vi "TrigNSave.vi"() -> ()   [LabVIEW 2013]
panel:
  in  "Trig Pulse Delay (s)":dbl[](array[numeric])
  in  "Trig Pulse Duration (s)":dbl[](array[numeric])
  in  "Delay between iterations (max exposure, in milliseconds)":i32=2000
  in  "Overwrite":bool
  in  "Save Data":bool
  out "Message":string
  in  "Pulse Energy mJ":dbl=5.0
  in  "File Name":string="log.dat"
  in  "Shot Num":i32
  in  "Shoot Once":bool
  in  "Abort Loop":bool
  out "Looping":bool
  out "Current Shot Number":i32
  in  "Number of shots":i32
  in  "START":bool
  in  "Command":string=":PULSe0:STATe ON"
  in  "Pressure reading mA":dbl=5.0
  in  "Pressure reading bar-a":dbl=1.0
  in  "Pulse Duration fs":dbl=5.0
  in  "Path to Folder":path=path "G:/Développement de Programmes/Programmes/octo-labview/Automatisation Manip Gaz"
  in  "Comments":string
  in  "FLSH":bool
  in  "SEND":bool
  out "error out":errorcluster
  in  "stop":bool
  out "read buffer":string
  in  "error in (no error)":errorcluster
  in  "VISA resource name":refnum<visa-resource-name>="COM1"
  # "Log File"
  # "Loop Control"
  # "BNC 505 Manual Control"
  # "Channel 0"
  # "Channel 1"
  # "Channel 2"
  # "Channel 3"
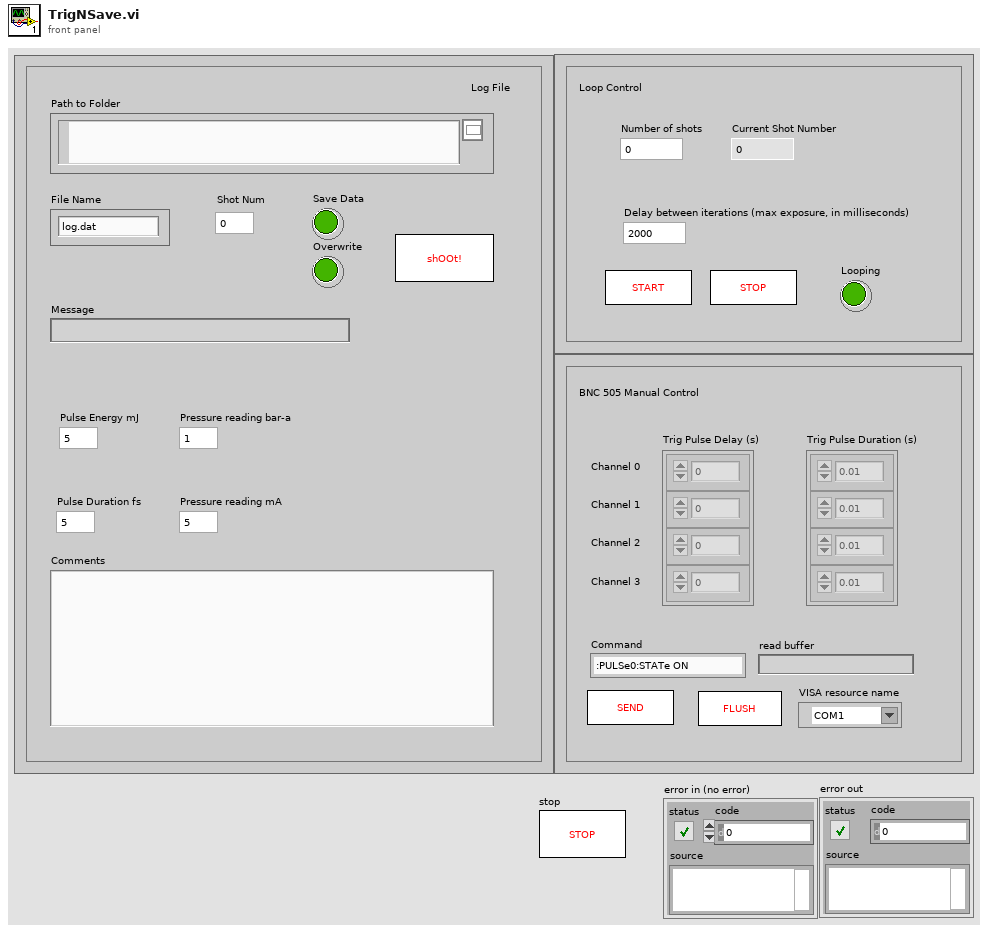
[diagram p1: front panel]
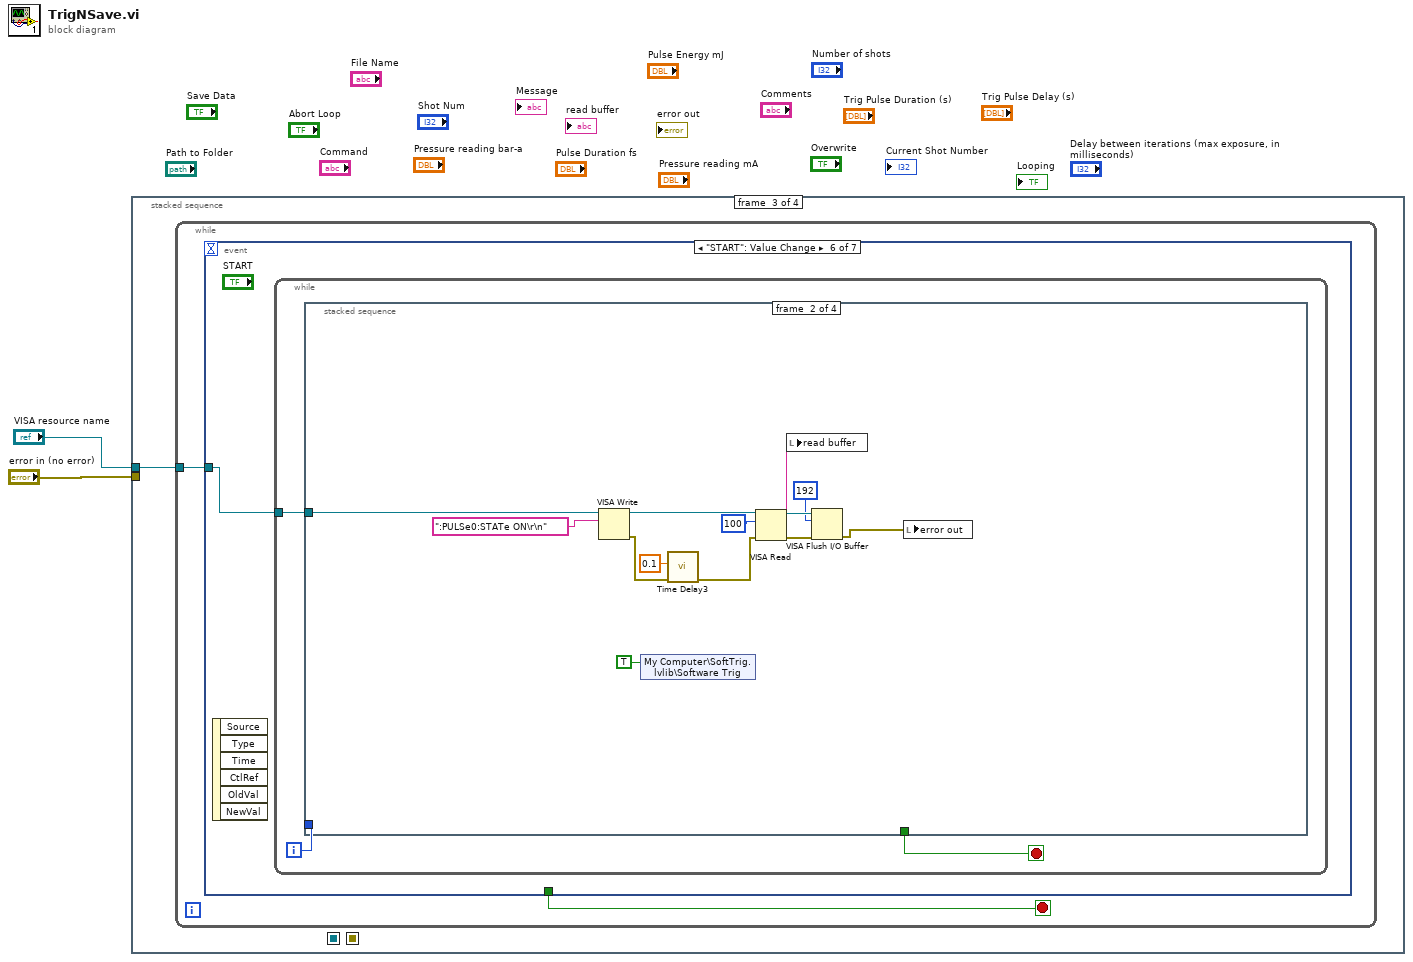
[diagram p0: block diagram]
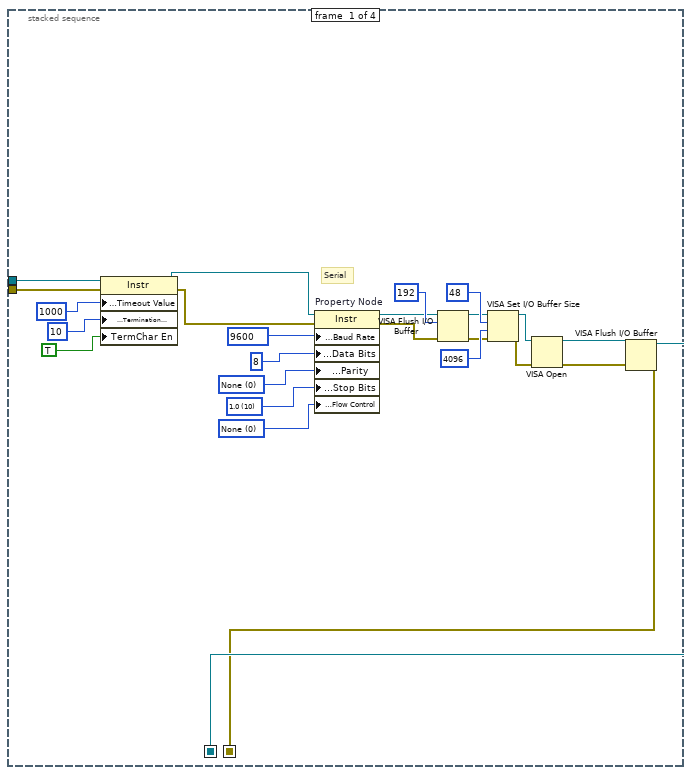
[diagram p2: hidden frame]
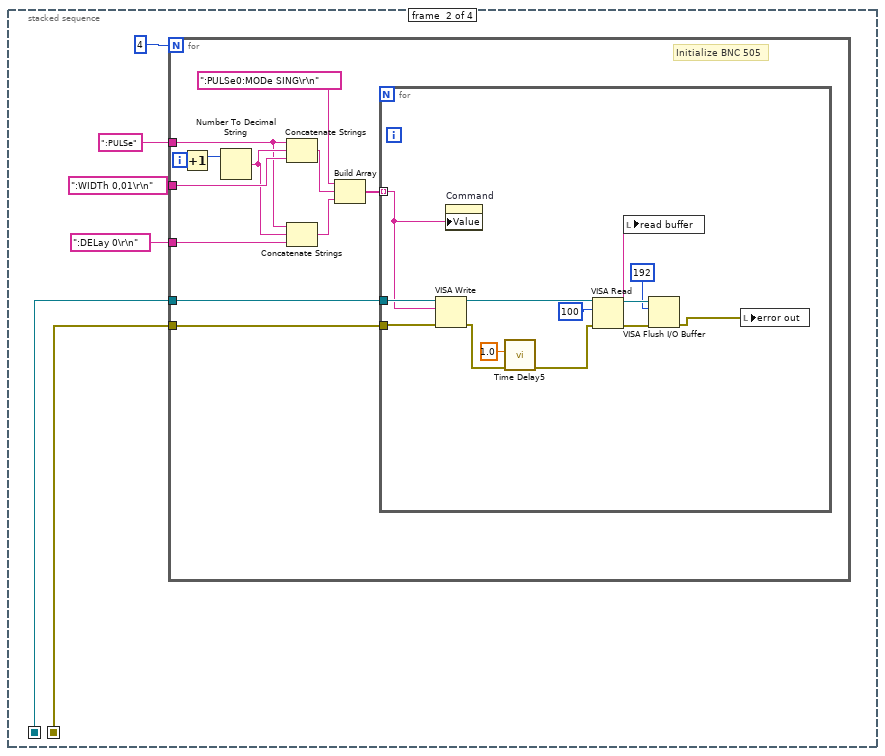
[diagram p3: hidden frame]
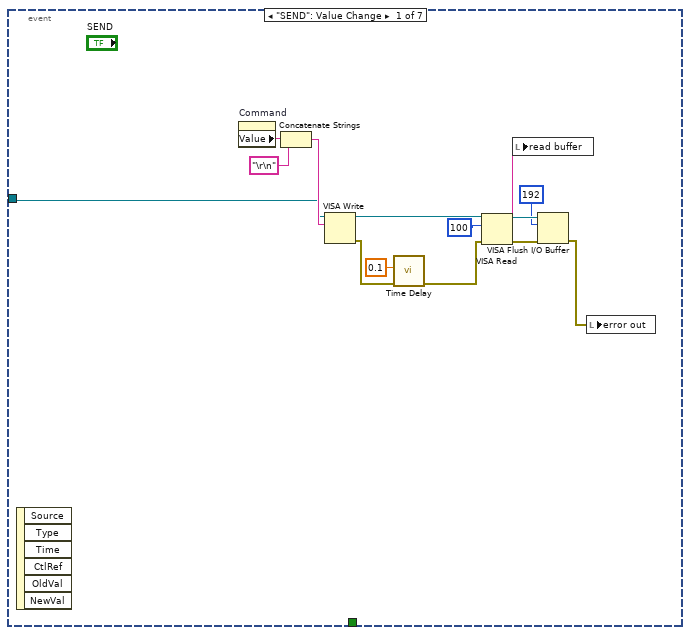
[diagram p4: hidden frame]
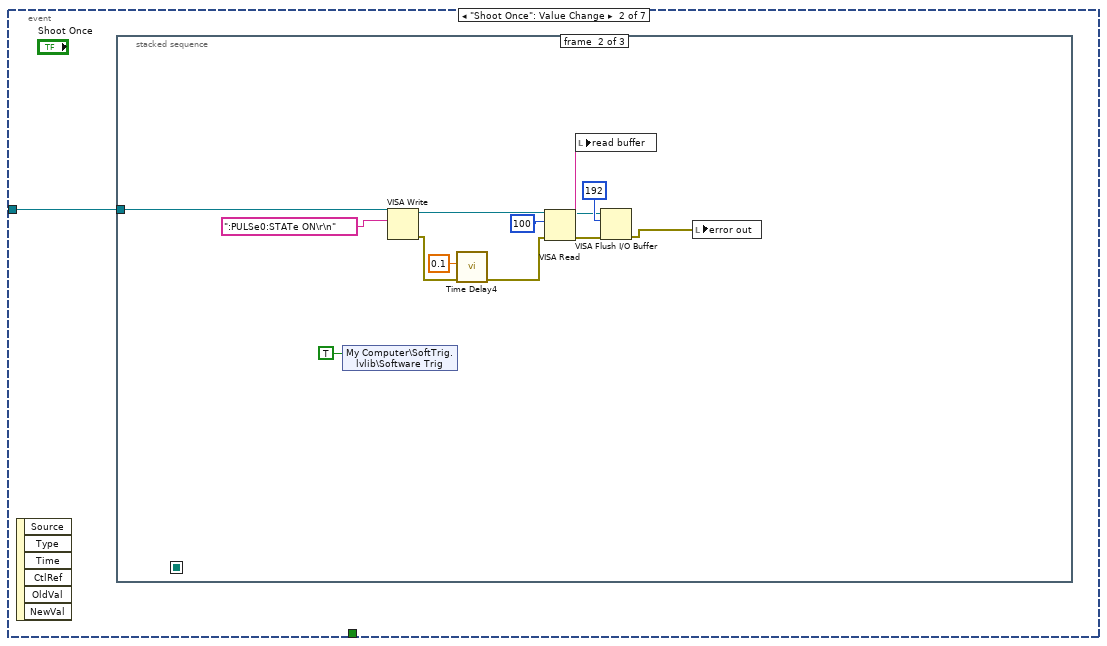
[diagram p5: hidden frame]
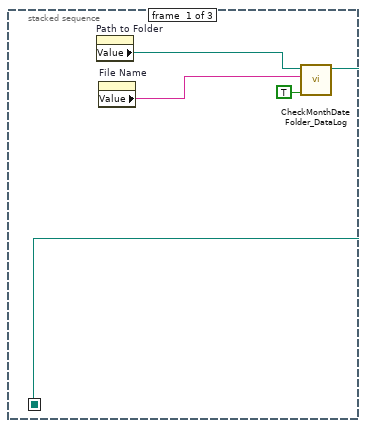
[diagram p6: hidden frame]
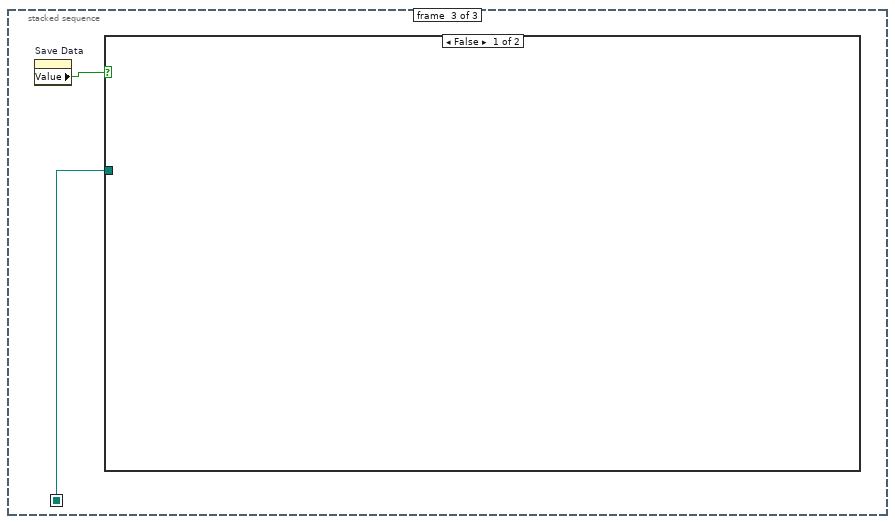
[diagram p7: hidden frame]
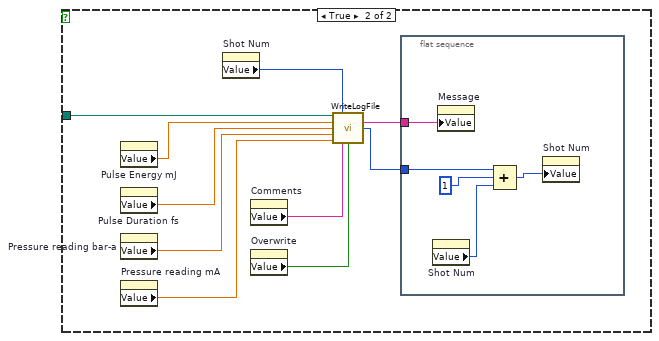
[diagram p8: hidden frame]
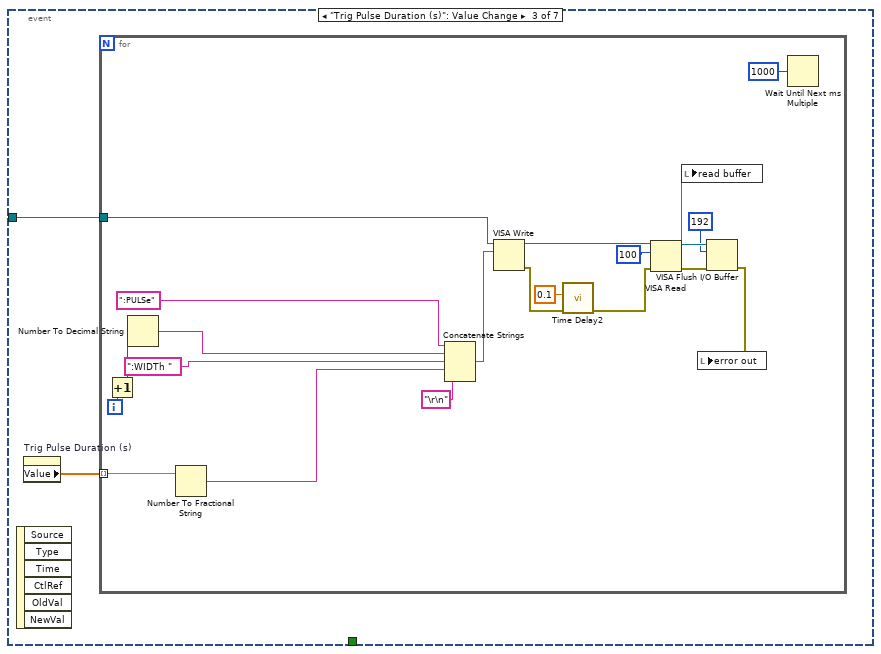
[diagram p9: hidden frame]
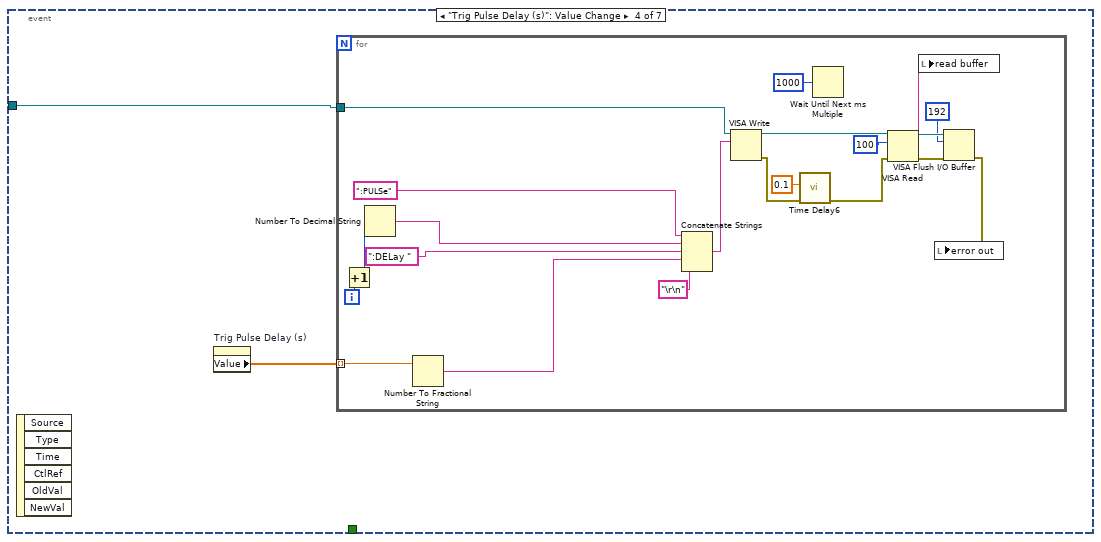
[diagram p10: hidden frame]
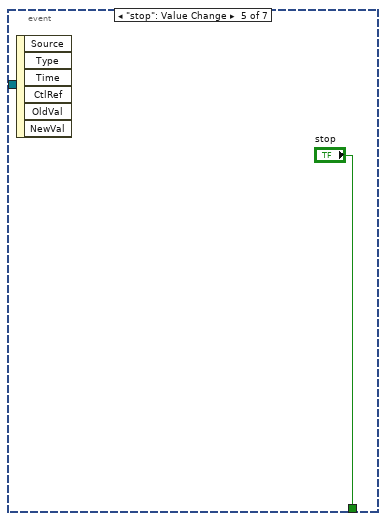
[diagram p11: hidden frame]
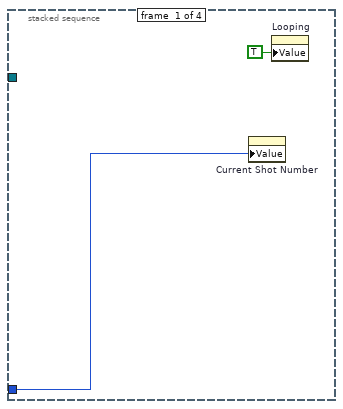
[diagram p12: hidden frame]
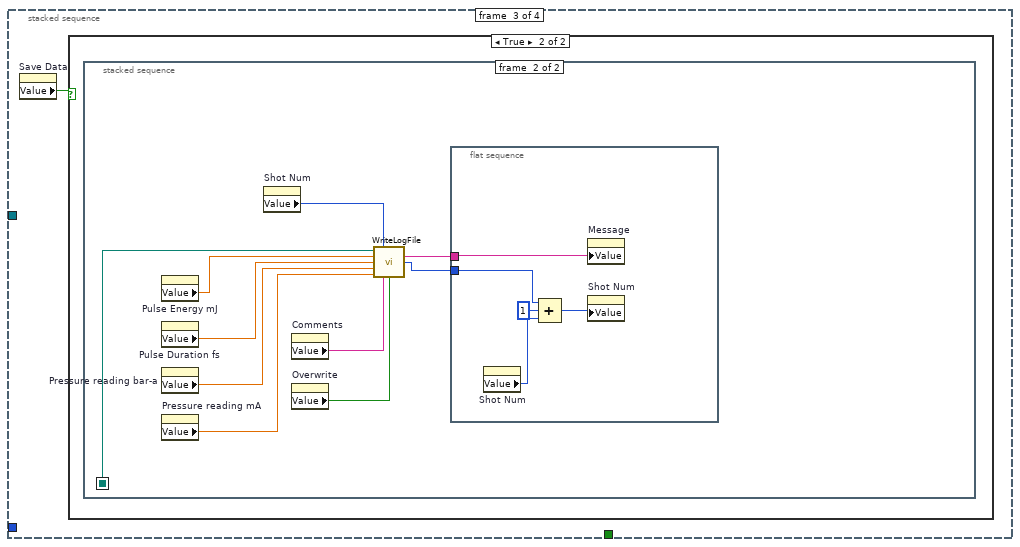
[diagram p13: hidden frame]
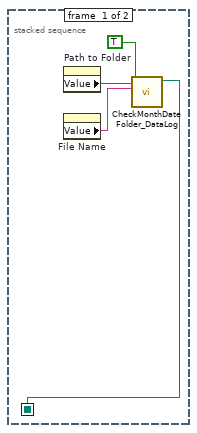
[diagram p15: hidden frame]
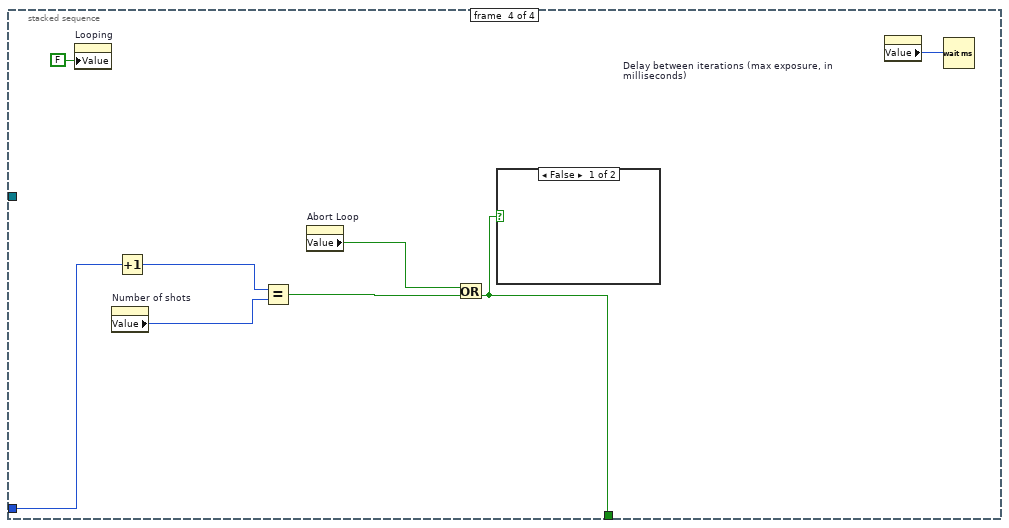
[diagram p16: hidden frame]
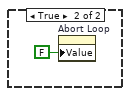
[diagram p17: hidden frame]
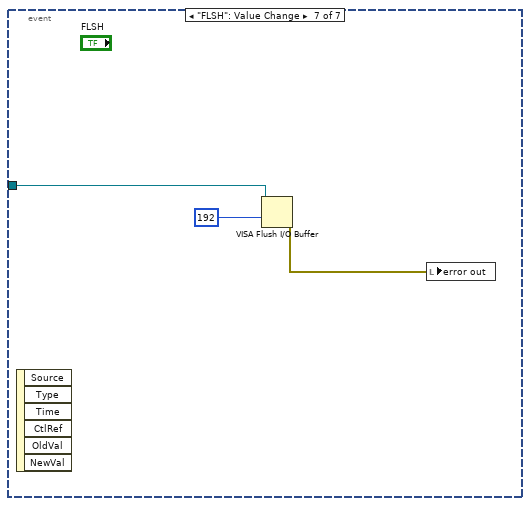
[diagram p18: hidden frame]
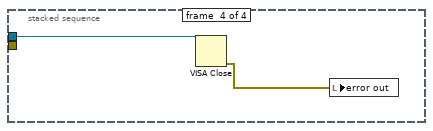
[diagram p19: hidden frame]
diagram:
  n1 = stacked-sequence {
    seq-local: [w4 _ _ _] -> [_ w33 _ _]
    seq-local: [w3 _ _ _] -> [_ w32 _ _]
    tunnel: "error in (no error)" -> [w22 _ _ _]
    tunnel: "VISA resource name" -> [w5 _ w59 w210]
    frame #0 {
      w11 = u32 9600 items=["4800"=4600, "9600"=9600, "19200"=19200, "38400"=38400, "57600"=57600, "115200"=115200] ("Baud Rate (make sure matches instrument)")
      w8 = u16 0 items=["None"=0, "XON/XOFF"=1, "RTS/CTS"=2, "DTR/DSR"=4] ("Serial Settings:Serial Flow Control")
      w19 = u16 10 items=["1.0"=10, "1.5"=15, "2.0"=20] ("Serial Settings:Serial Stop Bits")
      w20 = u16 0 items=["None", "Odd", "Even", "Mark", "Space"] ("Serial Settings:Serial Parity")
      # "Serial"
      n2 = property class="Instr"(reference=w5, error in=w22, "General Settings:Timeout Value"=u32 1000, "Message Based Settings:Termination Character"=u8 10, "TermChar En"=TRUE ("Message Based Settings:Termination Character Enable")) -> (reference out=w9:refnum<visa-resource-name>, error out=w10:errorcluster)
      n3 = property on="Property Node" class="Instr"(reference=w9, error in=w10, "Serial Settings:Baud Rate"=w11, "Serial Settings:Data Bits"=u16 8 ("Serial Settings:Serial Data Bits"), "Serial Settings:Parity"=w20, "Serial Settings:Stop Bits"=w19, "Serial Settings:Flow Control"=w8) -> (reference out=w13:refnum<visa-resource-name>, error out=w12:errorcluster)
      n4 = VISA Flush I/O Buffer(VISA resource name=w13, mask (16)=u16 192, error in (no error)=w12) -> (VISA resource name out=w14:refnum<visa-resource-name>, error out=w15:errorcluster)
      n5 = VISA Set I/O Buffer Size(VISA resource name=w14, mask (16)=u16 48, size (4096)=u32 4096 ("size (0)"), error in (no error)=w15) -> (VISA resource name out=w7:refnum<visa-resource-name>, error out=w6:errorcluster)
      n6 = VISA Open(error in (no error)=w6, VISA resource name=w7) -> (VISA resource name=w27:refnum<visa-resource-name>, error out=w26:errorcluster)  [unwired: 3 in]
      n7 = VISA Flush I/O Buffer(VISA resource name=w27, error in (no error)=w26) -> (VISA resource name out=w4:refnum<visa-resource-name>, error out=w3:errorcluster)  [unwired: 1 in]
    }
    frame #1 {
      n8 = for {
        N: 4 -> [_]
        tunnel: w33 -> [w45]
        tunnel: w32 -> [w44]
        tunnel: ":PULSe" ("write buffer") -> [w35]
        tunnel: ":WIDTh 0,01\r\n" ("write buffer") -> [w42]
        tunnel: ":DELay 0\r\n" ("write buffer") -> [w38]
        i -> [w43]
        # "Initialize BNC 505"
        n9 = Increment(x=w43) -> (x+1=w34:i32)
        n10 = Number To Decimal String(number=w34) -> (decimal integer string=w39:string)  [unwired: 1 in]
        n11 = Concatenate Strings(w35, w39, w42) -> (w40:string)
        n12 = Concatenate Strings(w35, w39, w38) -> (w37:string)
        n13 = Build Array(":PULSe0:MODe SING\r\n" ("write buffer"), w40, w37) -> (w36:string[])
        n14 = for {
          tunnel: w45 -> [w48]
          tunnel: w44 -> [w47]
          tunnel: w36 -> [w46] mode=indexing
          n15 = VISA Write(VISA resource name=w48, write buffer=w46, error in (no error)=w47) -> (VISA resource name out=w58:refnum<visa-resource-name>, error out=w53:errorcluster)  [unwired: 1 out]
          n16 = property on="Command" class="Str"("Value"=w46) -> ()  [unwired: 2 in, 2 out]
          n17 = call "Time Delay5"("error in (no error)"=w53, "Delay Time (s)"=1.0) -> ("error out"=w52:errorcluster)  [unwired: 9 out]
          n18 = VISA Read(VISA resource name=w58, byte count=u32 100, error in (no error)=w52) -> (VISA resource name out=w56:refnum<visa-resource-name>, read buffer=w50:string, error out=w55:errorcluster)  [unwired: 1 out]
          n19 = local write "read buffer"(w50) -> ()
          n20 = VISA Flush I/O Buffer(VISA resource name=w56, mask (16)=u16 192, error in (no error)=w55) -> (error out=w49:errorcluster)  [unwired: 1 out]
          n21 = local write "error out"(w49) -> ()
        }
      }
    }
    frame #2 {
      n22 = while {
        tunnel: w59 -> [w60]
        stop <- w61 stop-if-true
        n23 = event shown="[5] \"START\": Value Change" {
          selector: _ -> [_ _ _ _ _ _ _]
          dyn-events: _ -> [_ _ _ _ _ _ _]
          timeout: _ -> [_ _ _ _ _ _ _]
          tunnel: [_ _ _ _ "stop" _ _] -> w61
          tunnel: w60 -> [w62 w76 w111 w135 _ w158 w207]
          event "SEND": Value Change {
            n24 = event-data() -> ()  [unwired: 1 in, 6 out]
            n25 = property on="Command" class="Str"() -> ("Value"=w63:string)  [unwired: 2 in, 2 out]
            n26 = Concatenate Strings(w63, "\r\n" ("string")) -> (w64:string)
            n27 = VISA Write(VISA resource name=w62, write buffer=w64) -> (VISA resource name out=w75:refnum<visa-resource-name>, error out=w70:errorcluster)  [unwired: 1 in, 1 out]
            n28 = call "Time Delay"("error in (no error)"=w70, "Delay Time (s)"=0.1) -> ("error out"=w69:errorcluster)  [unwired: 9 out]
            n29 = VISA Read(VISA resource name=w75, byte count=u32 100, error in (no error)=w69) -> (VISA resource name out=w73:refnum<visa-resource-name>, read buffer=w67:string, error out=w72:errorcluster)  [unwired: 1 out]
            n30 = local write "read buffer"(w67) -> ()
            n31 = VISA Flush I/O Buffer(VISA resource name=w73, mask (16)=u16 192, error in (no error)=w72) -> (error out=w66:errorcluster)  [unwired: 1 out]
            n32 = local write "error out"(w66) -> ()
          }
          event "Shoot Once": Value Change {
            n33 = event-data() -> ()  [unwired: 1 in, 6 out]
            n34 = stacked-sequence {
              seq-local: [w78 _ _] -> [_ _ w95]
              tunnel: w76 -> [_ w82 _]
              frame #0 {
                n35 = property on="Path to Folder" class="Path"() -> ("Value"=w80:path)  [unwired: 2 in, 2 out]
                n36 = property on="File Name" class="Str"() -> ("Value"=w79:string)  [unwired: 2 in, 2 out]
                n37 = call "CheckMonthDateFolder_DataLog.vi"("Overwrite?"=TRUE, "File Name"=w79, "Folder Path Control"=w80) -> ("File Path"=w78:path)  [unwired: 6 in, 2 out]
              }
              frame #1 {
                n38 = shared-variable "My Computer\\SoftTrig.lvlib\\Software Trig"(TRUE ("Software Trig")) -> ()  [unwired: 1 in, 1 out]
                n39 = VISA Write(VISA resource name=w82, write buffer=":PULSe0:STATe ON\r\n") -> (VISA resource name out=w83:refnum<visa-resource-name>, error out=w88:errorcluster)  [unwired: 1 in, 1 out]
                n40 = call "Time Delay4"("error in (no error)"=w88, "Delay Time (s)"=0.1) -> ("error out"=w89:errorcluster)  [unwired: 9 out]
                n41 = VISA Read(VISA resource name=w83, byte count=u32 100, error in (no error)=w89) -> (VISA resource name out=w85:refnum<visa-resource-name>, read buffer=w91:string, error out=w86:errorcluster)  [unwired: 1 out]
                n42 = local write "read buffer"(w91) -> ()
                n43 = VISA Flush I/O Buffer(VISA resource name=w85, mask (16)=u16 192, error in (no error)=w86) -> (error out=w92:errorcluster)  [unwired: 1 out]
                n44 = local write "error out"(w92) -> ()
              }
              frame #2 {
                n45 = property on="Save Data" class="Bool (strict)"() -> ("Value"=w94:bool)  [unwired: 2 in, 2 out]
                n46 = case shown="False" w94 {
                  tunnel: w95 -> [_ w97]
                  frame False {
                  }
                  frame True {
                    n47 = property on="Pulse Energy mJ" class="DigNum (strict)"() -> ("Value"=w104:dbl)  [unwired: 2 in, 2 out]
                    n48 = property on="Pulse Duration fs" class="DigNum (strict)"() -> ("Value"=w103:dbl)  [unwired: 2 in, 2 out]
                    n49 = property on="Pressure reading bar-a" class="DigNum (strict)"() -> ("Value"=w102:dbl)  [unwired: 2 in, 2 out]
                    n50 = property on="Pressure reading mA" class="DigNum (strict)"() -> ("Value"=w101:dbl)  [unwired: 2 in, 2 out]
                    n51 = property on="Shot Num" class="DigNum (strict)"() -> ("Value"=w105:i32)  [unwired: 2 in, 2 out]
                    n52 = property on="Comments" class="Str"() -> ("Value"=w100:string)  [unwired: 2 in, 2 out]
                    n53 = property on="Overwrite" class="Bool (strict)"() -> ("Value"=w99:bool)  [unwired: 2 in, 2 out]
                    n54 = call "WriteLogFile.vi"("Path to File"=w97, "Shot Num"=w105, "Pulse Energy fs"=w104, "Pulse Duration fs"=w103, "Pressure reading bar-a"=w102, "Pressure reading mA"=w101, "Comments"=w100, "Overwrite"=w99) -> ("Message"=w98:string, "Success?"=w96:i32)  [unwired: 6 in]
                    n55 = flat-sequence {
                      tunnel: w98 -> [w110]
                      tunnel: w96 -> [w109]
                      frame #0 {
                        n56 = property on="Shot Num" class="DigNum (strict)"() -> ("Value"=w107:i32)  [unwired: 2 in, 2 out]
                        n57 = property on="Message" class="Str"("Value"=w110) -> ()  [unwired: 2 in, 2 out]
                        n58 = Compound Arithmetic op=ADD(w109, 1, w107) -> (w106:i32)
                        n59 = property on="Shot Num" class="DigNum (strict)"("Value"=w106) -> ()  [unwired: 2 in, 2 out]
                      }
                    }
                  }
                }
              }
            }
          }
          event "Trig Pulse Duration (s)": Value Change {
            n60 = event-data() -> ()  [unwired: 1 in, 6 out]
            n61 = property on="Trig Pulse Duration (s)" class="Arr (strict)"() -> ("Value"=w112:dbl[])  [unwired: 2 in, 2 out]
            n62 = for {
              tunnel: w112 -> [w115] mode=indexing
              tunnel: w111 -> [w113]
              i -> [w120]
              n63 = Increment(x=w120) -> (x+1=w121:i32)
              n64 = Number To Decimal String(number=w121) -> (decimal integer string=w118:string)  [unwired: 1 in]
              n65 = Number To Fractional String(number=w115) -> (F-format string=w114:string)  [unwired: 3 in]
              n66 = Concatenate Strings(":PULSe" ("string"), w118, ":WIDTh " ("string"), w114, "\r\n" ("string")) -> (w122:string)
              n67 = VISA Write(VISA resource name=w113, write buffer=w122) -> (VISA resource name out=w133:refnum<visa-resource-name>, error out=w128:errorcluster)  [unwired: 1 in, 1 out]
              n68 = call "Time Delay2"("error in (no error)"=w128, "Delay Time (s)"=0.1) -> ("error out"=w127:errorcluster)  [unwired: 9 out]
              n69 = VISA Read(VISA resource name=w133, byte count=u32 100, error in (no error)=w127) -> (VISA resource name out=w131:refnum<visa-resource-name>, read buffer=w125:string, error out=w130:errorcluster)  [unwired: 1 out]
              n70 = local write "read buffer"(w125) -> ()
              n71 = VISA Flush I/O Buffer(VISA resource name=w131, mask (16)=u16 192, error in (no error)=w130) -> (error out=w124:errorcluster)  [unwired: 1 out]
              n72 = local write "error out"(w124) -> ()
              n73 = Wait Until Next ms Multiple(millisecond multiple=u32 1000) -> ()  [unwired: 1 out]
            }
          }
          event "Trig Pulse Delay (s)": Value Change {
            n74 = event-data() -> ()  [unwired: 1 in, 6 out]
            n75 = property on="Trig Pulse Delay (s)" class="Arr (strict)"() -> ("Value"=w134:dbl[])  [unwired: 2 in, 2 out]
            n76 = for {
              tunnel: w134 -> [w138] mode=indexing
              tunnel: w135 -> [w136]
              i -> [w143]
              n77 = Increment(x=w143) -> (x+1=w144:i32)
              n78 = Number To Decimal String(number=w144) -> (decimal integer string=w141:string)  [unwired: 1 in]
              n79 = Number To Fractional String(number=w138) -> (F-format string=w137:string)  [unwired: 3 in]
              n80 = Concatenate Strings(":PULSe" ("string"), w141, ":DELay " ("string"), w137, "\r\n" ("string")) -> (w145:string)
              n81 = VISA Write(VISA resource name=w136, write buffer=w145) -> (VISA resource name out=w156:refnum<visa-resource-name>, error out=w151:errorcluster)  [unwired: 1 in, 1 out]
              n82 = call "Time Delay6"("error in (no error)"=w151, "Delay Time (s)"=0.1) -> ("error out"=w150:errorcluster)  [unwired: 9 out]
              n83 = Wait Until Next ms Multiple(millisecond multiple=u32 1000) -> ()  [unwired: 1 out]
              n84 = VISA Read(VISA resource name=w156, byte count=u32 100, error in (no error)=w150) -> (VISA resource name out=w154:refnum<visa-resource-name>, read buffer=w148:string, error out=w153:errorcluster)  [unwired: 1 out]
              n85 = local write "read buffer"(w148) -> ()
              n86 = VISA Flush I/O Buffer(VISA resource name=w154, mask (16)=u16 192, error in (no error)=w153) -> (error out=w147:errorcluster)  [unwired: 1 out]
              n87 = local write "error out"(w147) -> ()
            }
          }
          event "stop": Value Change {
            n88 = event-data() -> ()  [unwired: 1 in, 6 out]
          }
          event "START": Value Change {
            n89 = event-data() -> ()  [unwired: 1 in, 6 out]
            n90 = while {
              tunnel: w158 -> [w159]
              i -> [w161]
              stop <- w160 stop-if-true
              n91 = stacked-sequence {
                tunnel: w161 -> [w163 _ _ w204]
                tunnel: [_ _ _ w199] -> w160
                tunnel: w159 -> [_ w166 _ _]
                frame #0 {
                  n92 = property on="Current Shot Number" class="DigNum (strict)"("Value"=w163) -> ()  [unwired: 2 in, 2 out]
                  n93 = property on="Looping" class="Bool (strict)"("Value"=TRUE ("Looping")) -> ()  [unwired: 2 in, 2 out]
                }
                frame #1 {
                  n94 = VISA Write(VISA resource name=w166, write buffer=":PULSe0:STATe ON\r\n") -> (VISA resource name out=w176:refnum<visa-resource-name>, error out=w171:errorcluster)  [unwired: 1 in, 1 out]
                  n95 = shared-variable "My Computer\\SoftTrig.lvlib\\Software Trig"(TRUE ("Software Trig")) -> ()  [unwired: 1 in, 1 out]
                  n96 = call "Time Delay3"("error in (no error)"=w171, "Delay Time (s)"=0.1) -> ("error out"=w170:errorcluster)  [unwired: 9 out]
                  n97 = VISA Read(VISA resource name=w176, byte count=u32 100, error in (no error)=w170) -> (VISA resource name out=w174:refnum<visa-resource-name>, read buffer=w168:string, error out=w173:errorcluster)  [unwired: 1 out]
                  n98 = local write "read buffer"(w168) -> ()
                  n99 = VISA Flush I/O Buffer(VISA resource name=w174, mask (16)=u16 192, error in (no error)=w173) -> (error out=w167:errorcluster)  [unwired: 1 out]
                  n100 = local write "error out"(w167) -> ()
                }
                frame #2 {
                  n101 = property on="Save Data" class="Bool (strict)"() -> ("Value"=w177:bool)  [unwired: 2 in, 2 out]
                  n102 = case shown="True" w177 {
                    frame False {
                    }
                    frame True {
                      n103 = stacked-sequence {
                        seq-local: [w178 _] -> [_ w191]
                        frame #0 {
                          n104 = property on="Path to Folder" class="Path"() -> ("Value"=w181:path)  [unwired: 2 in, 2 out]
                          n105 = property on="File Name" class="Str"() -> ("Value"=w180:string)  [unwired: 2 in, 2 out]
                          n106 = call "CheckMonthDateFolder_DataLog.vi"("Overwrite?"=TRUE, "File Name"=w180, "Folder Path Control"=w181) -> ("File Path"=w178:path)  [unwired: 6 in, 2 out]
                        }
                        frame #1 {
                          n107 = property on="Pulse Energy mJ" class="DigNum (strict)"() -> ("Value"=w189:dbl)  [unwired: 2 in, 2 out]
                          n108 = property on="Pulse Duration fs" class="DigNum (strict)"() -> ("Value"=w188:dbl)  [unwired: 2 in, 2 out]
                          n109 = property on="Pressure reading bar-a" class="DigNum (strict)"() -> ("Value"=w187:dbl)  [unwired: 2 in, 2 out]
                          n110 = property on="Pressure reading mA" class="DigNum (strict)"() -> ("Value"=w186:dbl)  [unwired: 2 in, 2 out]
                          n111 = property on="Shot Num" class="DigNum (strict)"() -> ("Value"=w190:i32)  [unwired: 2 in, 2 out]
                          n112 = property on="Comments" class="Str"() -> ("Value"=w185:string)  [unwired: 2 in, 2 out]
                          n113 = property on="Overwrite" class="Bool (strict)"() -> ("Value"=w184:bool)  [unwired: 2 in, 2 out]
                          n114 = call "WriteLogFile.vi"("Path to File"=w191, "Shot Num"=w190, "Pulse Energy fs"=w189, "Pulse Duration fs"=w188, "Pressure reading bar-a"=w187, "Pressure reading mA"=w186, "Comments"=w185, "Overwrite"=w184) -> ("Message"=w183:string, "Success?"=w182:i32)  [unwired: 6 in]
                          n115 = flat-sequence {
                            tunnel: w183 -> [w196]
                            tunnel: w182 -> [w193]
                            frame #0 {
                              n116 = property on="Shot Num" class="DigNum (strict)"() -> ("Value"=w195:i32)  [unwired: 2 in, 2 out]
                              n117 = Compound Arithmetic op=ADD(w193, 1 ("value"), w195) -> (w192:i32)
                              n118 = property on="Message" class="Str"("Value"=w196) -> ()  [unwired: 2 in, 2 out]
                              n119 = property on="Shot Num" class="DigNum (strict)"("Value"=w192) -> ()  [unwired: 2 in, 2 out]
                            }
                          }
                        }
                      }
                    }
                  }
                }
                frame #3 {
                  n120 = property on="Looping" class="Bool (strict)"("Value"=FALSE ("Looping")) -> ()  [unwired: 2 in, 2 out]
                  n121 = property on="Number of shots" class="DigNum (strict)"() -> ("Value"=w203:i32)  [unwired: 2 in, 2 out]
                  n122 = Increment(x=w204) -> (x+1=w201:i32)
                  n123 = Equal?(x=w201, y=w203) -> (x = y?=w202:bool)
                  n124 = property on="Abort Loop" class="Bool (strict)"() -> ("Value"=w200:bool)  [unwired: 2 in, 2 out]
                  n125 = Or(x=w200, y=w202) -> (x .or. y?=w199:bool)
                  n126 = case shown="False" w199 {
                    frame False {
                    }
                    frame True {
                      n127 = property on="Abort Loop" class="Bool (strict)"("Value"=FALSE ("Abort Loop")) -> ()  [unwired: 2 in, 2 out]
                    }
                  }
                  n128 = property on="Delay between iterations (max exposure, in milliseconds)" class="DigNum (strict)"() -> ("Value"=w197:i32)  [unwired: 2 in, 2 out]
                  n129 = Wait (ms)(milliseconds to wait=w197) -> ()  [unwired: 1 out]
                }
              }
            }
          }
          event "FLSH": Value Change {
            n130 = event-data() -> ()  [unwired: 1 in, 6 out]
            n131 = VISA Flush I/O Buffer(VISA resource name=w207, mask (16)=u16 192) -> (error out=w206:errorcluster)  [unwired: 1 in, 1 out]
            n132 = local write "error out"(w206) -> ()
          }
        }
      }
    }
    frame #3 {
      n133 = VISA Close(VISA resource name=w210) -> (error out=w209:errorcluster)  [unwired: 1 in]
      n134 = local write "error out"(w209) -> ()
    }
  }
